vi "Projectile.vi"() -> ()   [LabVIEW 2014]
uses:
  <vilib>/imath/engines/lvmath2/RunTimeEngine/Managers/WorkSpace/UID Generator.vi
  <vilib>/imath/engines/lvmath2/RunTimeEngine/RunTimeType/NIMS_RunTimeType_From StrictType (excl LVString).vi
  <instcachedir>/0/NIMS_RunTimeType_From StrictType (excl LVString)_15A5391EEA9C4AACB9955AC755B83D29.lvgen/NIMS_RunTimeType_From StrictType (excl LVString)_15A5391EEA9C4AACB9955AC755B83D29_000.vi
  <vilib>/imath/engines/lvmath2/RunTimeEngine/LocalVariableDefStatement/MC_LocalVariableDefStatement_Display.vi
  <vilib>/imath/engines/lvmath2/RunTimeEngine/Managers/SymbolTable/Clear UID.vi
  <vilib>/imath/engines/lvmath2/RunTimeEngine/NodeEndStatement/NIMS_NodeEndStatement_Output.vi
  <instcachedir>/0/NIMS_NodeEndStatement_Output_53EC0D466D134D7ABD903AC30B43404B.lvgen/NIMS_NodeEndStatement_Output_53EC0D466D134D7ABD903AC30B43404B_005.vi
  <instcachedir>/0/NIMS_NodeEndStatement_Output_53EC0D466D134D7ABD903AC30B43404B.lvgen/NIMS_NodeEndStatement_Output_53EC0D466D134D7ABD903AC30B43404B_004.vi
  <vilib>/imath/engines/lvmath2/RunTimeEngine/ErrorHandling/NIMS_Finalize Error.vi
  <vilib>/imath/engines/lvmath2/RunTimeEngine/Managers/SymbolTable/NIMS_WorkSpace.lvlib
panel:
  out "output cluster":cluster{"theta":dbl[], "R":dbl[]}
  out "XY Graph":cluster{"theta":i32[], "R":dbl[]}(graph)
  in  "Launch Height (m)":dbl
  in  "Launch Speed (m/s)":dbl
  # "ANSWERS. \nC. angle that produces maximum range at height\n2.1 meters is 42 degrees\nD. ange that produces maximum range at height\n100 meters is 16 degrees"
  # "The display shows the range a projectile will have at different launch angles\n(0 through 90 degrees) given a user specified launch speed and launch height."
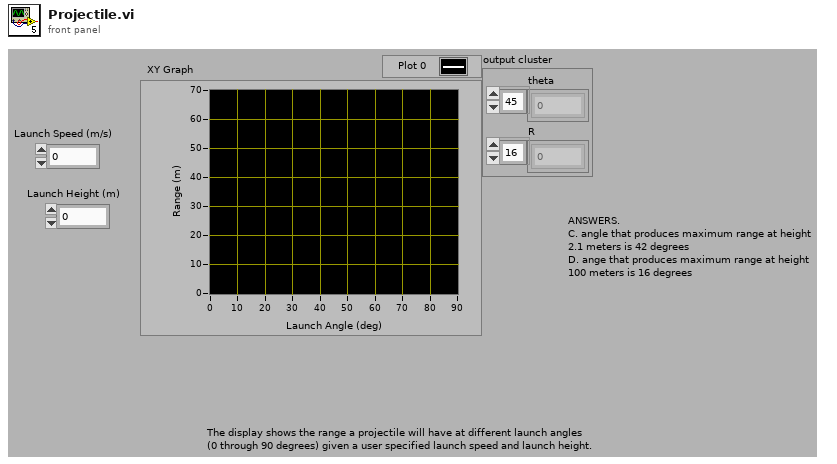
[diagram p1: front panel]
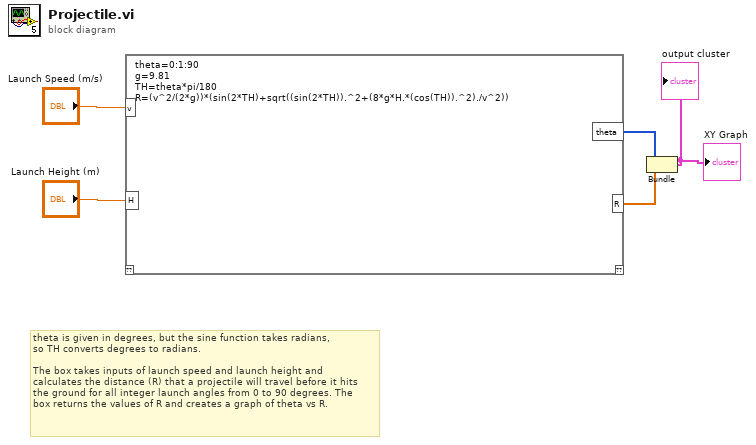
[diagram p0: block diagram]
diagram:
  # "theta is given in degrees, but the sine function takes radians,\nso TH converts degrees to radians.\n\nThe box takes inputs of launch speed and launch height and\ncalculates the distance (R) that a projectile will travel before it hits\nthe ground for all integer launch angles from 0 to 90 degrees. The\nbox returns the values of R and creates a graph of theta vs R."
  n1 = mathscript code="theta=0:1:90\ng=9.81\nTH=theta*pi/180\nR=(v^2/(2*g))*(sin(2*TH)+sqrt((sin(2*TH)).^2+(8*g*H.*(cos(TH)).^2)./v^2))"("v"="Launch Speed (m/s)", "H"="Launch Height (m)") -> ("theta"=w5:i32[], "R"=w4:dbl[])  [unwired: 1 in, 1 out]
  n2 = Bundle("theta"=w5, "R"=w4) -> (→"XY Graph" →"output cluster":cluster{"theta":i32[], "R":dbl[]})  [unwired: 1 in]
